vi "Client tcpip.vi"(0 "Type of wash":string, 1 "Time":string, 2 "Date":string) -> ()   [LabVIEW 2021]
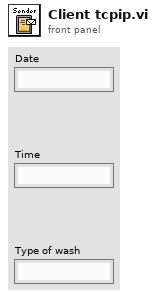
[diagram p1: front panel]
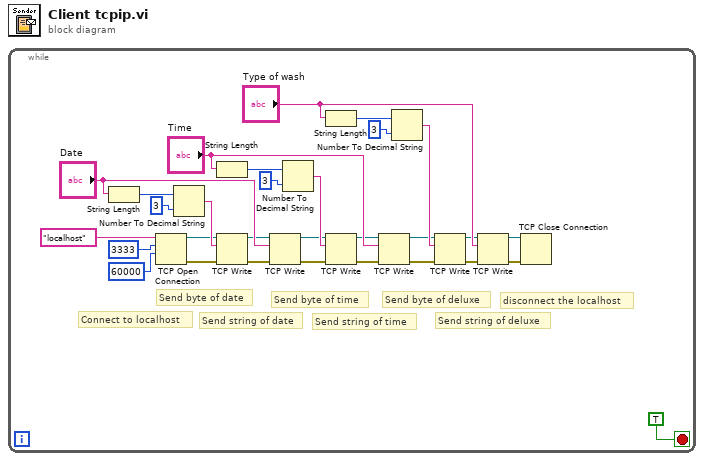
[diagram p0: block diagram]
diagram:
  n1 = while {
    stop <- TRUE stop-if-true
    # "disconnect the localhost"
    # "Send string of deluxe"
    # "Send byte of deluxe"
    # "Send string of time"
    # "Send byte of time"
    # "Send string of date"
    # "Send byte of date"
    # "Connect to localhost"
    n2 = String Length(string="Date") -> (length=w17:i32)
    n3 = TCP Open Connection(address="localhost", remote port or service name=u16 3333, timeout ms (60000)=60000) -> (connection ID=w5:refnum<k5>, error out=w6:errorcluster)  [unwired: 2 in]
    n4 = Number To Decimal String(number=w17, width (-)=i16 3) -> (decimal integer string=w19:string)
    n5 = String Length(string="Time") -> (length=w22:i32)
    n6 = TCP Write(connection ID=w5, data in=w19, error in (no error)=w6) -> (connection ID out=w7:refnum<k5>, error out=w8:errorcluster)  [unwired: 1 in, 1 out]
    n7 = TCP Write(connection ID=w7, data in="Date", error in (no error)=w8) -> (connection ID out=w9:refnum<k5>, error out=w10:errorcluster)  [unwired: 1 in, 1 out]
    n8 = Number To Decimal String(number=w22, width (-)=i16 3) -> (decimal integer string=w23:string)
    n9 = String Length(string="Type of wash") -> (length=w28:i32)
    n10 = TCP Write(connection ID=w9, data in=w23, error in (no error)=w10) -> (connection ID out=w11:refnum<k5>, error out=w12:errorcluster)  [unwired: 1 in, 1 out]
    n11 = TCP Write(connection ID=w11, data in="Time", error in (no error)=w12) -> (connection ID out=w13:refnum<k5>, error out=w14:errorcluster)  [unwired: 1 in, 1 out]
    n12 = Number To Decimal String(number=w28, width (-)=i16 3) -> (decimal integer string=w29:string)
    n13 = TCP Write(connection ID=w13, data in=w29, error in (no error)=w14) -> (connection ID out=w15:refnum<k5>, error out=w16:errorcluster)  [unwired: 1 in, 1 out]
    n14 = TCP Write(connection ID=w15, data in="Type of wash", error in (no error)=w16) -> (connection ID out=w25:refnum<k5>, error out=w26:errorcluster)  [unwired: 1 in, 1 out]
    n15 = TCP Close Connection(connection ID=w25, error in (no error)=w26) -> ()  [unwired: 1 in, 2 out]
  }
